vi "Read properties.vi"(11 "TestManagerMsg.Test in":refnum<class "TestManagerMsg.Test.lvclass">) -> (2 "properties":refnum<class "TestManagerMsg.KVP.lvclass">[](array[class]), 3 "TestManagerMsg.Test out":refnum<class "TestManagerMsg.Test.lvclass">)   [LabVIEW 2020, in "Caraya.lvlib" / "TestManagerMsg.Test.lvclass"]
uses:
  TestManagerMsg.Test.lvclass
  Test Manager Message KVP/TestManagerMsg.KVP.lvclass
  TestManagerMsg.Test.lvclass/TestManagerMsg.Test.ctl
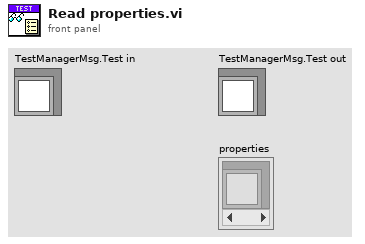
[diagram p1: front panel]
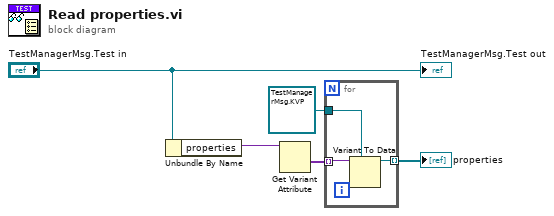
[diagram p0: block diagram]
diagram:
  n1 = Unbundle By Name("TestManagerMsg.Test in") -> ("properties"=w4:variant)
  n2 = Get Variant Attribute(Variant=w4) -> (values=w3:variant[])  [unwired: 3 in, 3 out]
  n3 = for {
    tunnel: w3 -> [w8] mode=indexing
    tunnel: refnum<class "TestManagerMsg.KVP.lvclass"> refnum ("KVP") -> [w7]
    tunnel: [w6] -> w1 mode=indexing
    n4 = Variant To Data(type=w7, Variant=w8) -> (data=w6:refnum<class "TestManagerMsg.KVP.lvclass">)  [unwired: 1 in, 1 out]
  }
  "properties" <- w1
  "TestManagerMsg.Test out" <- "TestManagerMsg.Test in"
